vi "Check Command is Valid.vi"(8 "error in":errorcluster, 9 "Cmd Sent":string, 10 "Cmd Response":string) -> (0 "error out":errorcluster, 2 "Cmd Response Out":string)   [LabVIEW 2019, in "Mercury iXX.lvlib"]
uses:
  Mercury iXX.lvlib
  <vilib>/regexp/Match Regular Expression.xnode
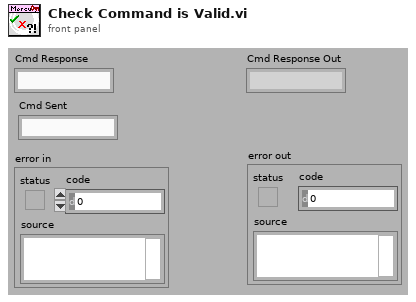
[diagram p1: front panel]
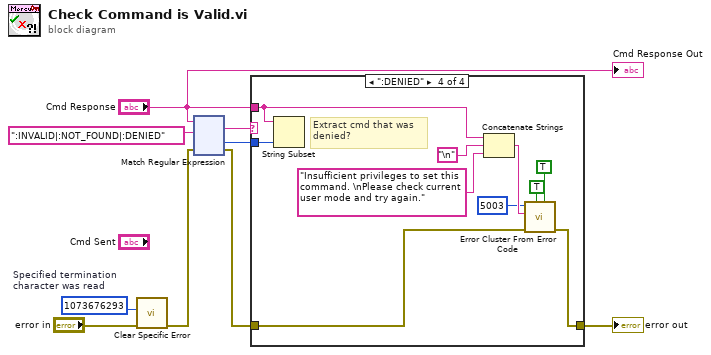
[diagram p0: block diagram]
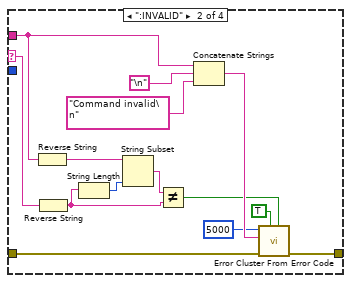
[diagram p3: hidden frame]
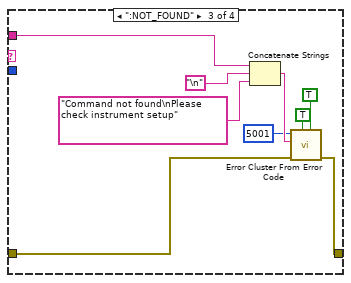
[diagram p4: hidden frame]
diagram:
  w1 = 1073676293  # Specified termination character was read
  n1 = call "Clear Specific Error.vi"("error in"="error in", "Code (-1:All)"=w1) -> ("error out"=w2:errorcluster)  [unwired: 9 out]
  n2 = xnode "Match Regular Expression"("input string"="Cmd Response", "regular expression"=":INVALID|:NOT_FOUND|:DENIED", "error in"=w2) -> ("whole match"=w7:string, "offset past match"=w5:i32, "error out"=w4:errorcluster)  [unwired: 1 in, 4 out]
  n3 = case shown="\":DENIED\"" w7 {
    selector: w7 -> [_ w16 _ _]
    tunnel: "Cmd Response" -> [_ w17 w25 w34]
    tunnel: [w10 w21 w30 w40] -> w8
    tunnel: w4 -> [w10 w20 w29 w39]
    tunnel: w5 -> [_ _ _ w35]
    frame "", Default {
    }
    frame ":INVALID" {
      n4 = Reverse String(1:w17) -> (0:w14:string)
      n5 = Reverse String(1:w16) -> (0:w12:string)
      n6 = String Length(string=w12) -> (length=w15:i32)
      n7 = String Subset(string=w14, length (rest)=w15) -> (substring=w13:string)  [unwired: 1 out]
      n8 = Not Equal?(x=w13, y=w12) -> (x != y?=w11:bool)
      n9 = Concatenate Strings(w17, "\n", "Command invalid\n" ("string")) -> (w24:string)
      n10 = call <vilib>:"Error Cluster From Error Code.vi"("is warning? (False)"=w11, "show call chain? (False)"=TRUE, "error in (no error)"=w20, "error message (\"\")"=w24, "error code (0)"=5000) -> ("error out"=w21:errorcluster)  [unwired: 4 out]
    }
    frame ":NOT_FOUND" {
      n11 = Concatenate Strings(w25, "\n", "Command not found\nPlease check instrument setup" ("string")) -> (w33:string)
      n12 = call <vilib>:"Error Cluster From Error Code.vi"("is warning? (False)"=TRUE, "show call chain? (False)"=TRUE, "error in (no error)"=w29, "error message (\"\")"=w33, "error code (0)"=5001) -> ("error out"=w30:errorcluster)  [unwired: 4 out]
    }
    frame ":DENIED" {
      # "Extract cmd that was \ndenied?"
      n13 = String Subset(string=w34, length (rest)=w35) -> ()  [unwired: 2 out]
      n14 = Concatenate Strings(w34, "\n", "Insufficient privileges to set this command. \nPlease check current user mode and try again." ("string")) -> (w43:string)
      n15 = call <vilib>:"Error Cluster From Error Code.vi"("is warning? (False)"=TRUE, "show call chain? (False)"=TRUE, "error in (no error)"=w39, "error message (\"\")"=w43, "error code (0)"=5003) -> ("error out"=w40:errorcluster)  [unwired: 4 out]
    }
  }
  "error out" <- w8
  "Cmd Response Out" <- "Cmd Response"
